vi "Gradient Read Single.vi"(8 "error in":errorcluster, 9 "Channel Index":i32=1, 11 "Pressure Gradient in":refnum<class "Pressure Gradient.lvclass">) -> (0 "error out":errorcluster, 1 "Changed or First Call?":bool, 2 "Pressure SP":dbl, 3 "Pressure Gradient out":refnum<class "Pressure Gradient.lvclass">)   [LabVIEW 2023, in "Pressure Gradient.lvclass"]
uses:
  Pressure Gradient.lvclass
  Parents/Gradient/Gradient.lvclass
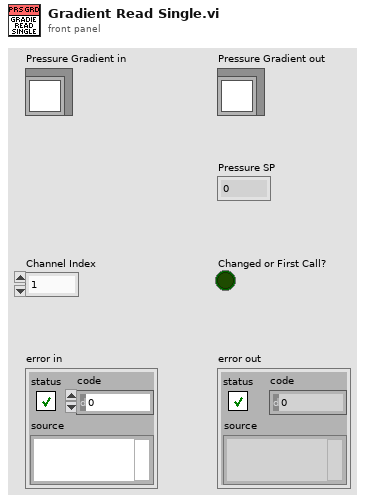
[diagram p1: front panel]
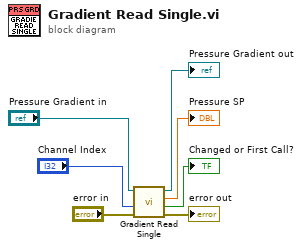
[diagram p0: block diagram]
diagram:
  n1 = call-parent "Gradient Read Single.vi"("error in"="error in", "Channel Index"="Channel Index", "Gradient in"="Pressure Gradient in") -> ("error out"=→"error out":errorcluster, "Changed or First Call?"=→"Changed or First Call?":bool, "Current SP"=→"Pressure SP":dbl, "Gradient out"=→"Pressure Gradient out":refnum<class "Pressure Gradient.lvclass">)  [unwired: 5 in]
